vi "Obtain Hwnd and instantiate.vi"(0 "Py Doc in":refnum<class "Py Doc.lvclass">, 11 "error in (no error)":errorcluster) -> (4 "Document Out":refnum<class "Document.lvclass">, 6 "Document out":refnum<class "Document.lvclass">, 15 "error out":errorcluster)   [LabVIEW 2016, in "Py Doc.lvclass"]
uses:
  Py Doc.lvclass
  D:/Navin Workspace/MDI/source code/Document/Document base/Document.lvclass
  Document base/Document.lvclass
  Document base/Document.lvclass/Document.ctl
  Child Classes/Py Editor/Py Editor.lvclass
  Child Classes/Py Shell/Py Shell.lvclass
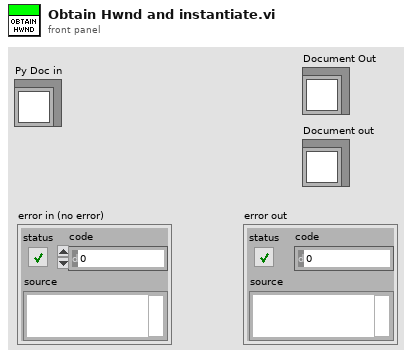
[diagram p1: front panel]
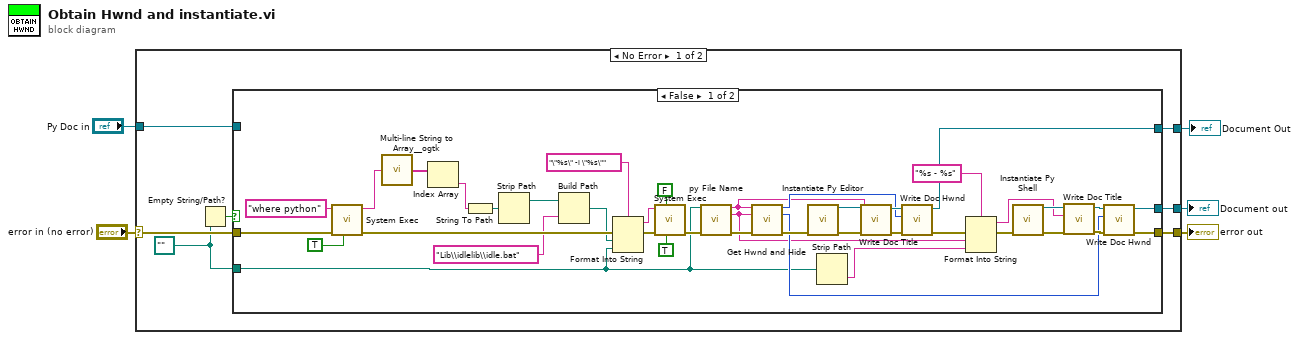
[diagram p0: block diagram]
diagram:
  n1 = case shown="No Error" "error in (no error)" {
    selector: "error in (no error)" -> [w11 w56]
    tunnel: "Py Doc in" -> [w10 w55]
    tunnel: [w12 w56] -> w4
    tunnel: [w8 w55] -> w2
    tunnel: [w7 w55] -> w1
    frame No Error {
      w6 = path "" ("Document Path")
      n2 = Empty String/Path?(string/path=w6) -> (empty?=w9:bool)
      n3 = case shown="False" w9 {
        tunnel: [w22 w54] -> w12
        tunnel: w11 -> [w35 w54]
        tunnel: w10 -> [_ w53]
        tunnel: w6 -> [w18 _]
        tunnel: [w20 w53] -> w8
        tunnel: [w19 w53] -> w7
        frame False {
          n4 = call <vilib>:"System Exec.vi"("run minimized? (F)"=TRUE, "error in (no error)"=w35, "command line"="where python") -> ("error out"=w52:errorcluster, "standard output"=w33:string)  [unwired: 5 in, 2 out]
          n5 = call <userlib>:"Multi-line String to Array__ogtk.vi"("string"=w33) -> ("lines"=w34:string[])
          n6 = Index Array(array=w34) -> (element=w32:string)  [unwired: 1 in]
          n7 = String To Path(string=w32) -> (path=w48:path)
          n8 = Strip Path(path=w48) -> (stripped path=w49:path)  [unwired: 1 out]
          n9 = Build Path(base path=w49, name or relative path="Lib\\idlelib\\idle.bat") -> (appended path=w51:path)
          n10 = Format Into String(format string="\"%s\" -i \"%s\"", error in=w52, w51, w18) -> (resulting string=w37:string, error out=w36:errorcluster)  [unwired: 1 in]
          n11 = call <vilib>:"System Exec.vi"("run minimized? (F)"=TRUE, "wait until completion? (T)"=FALSE, "error in (no error)"=w36, "command line"=w37) -> ("error out"=w42:errorcluster)  [unwired: 4 in, 3 out]
          n12 = call "py File Name.vi"("Path"=w18, "error in (no error)"=w42) -> ("Doc Name"=w43:string, "Shell Name"=w15:string, "error out"=w40:errorcluster)  [unwired: 11 in]
          n13 = call "Get Hwnd and Hide.vi"("Doc Name"=w43, "Shell Name"=w15, "error in (no error)"=w40) -> ("Child hwnd"=w44:u32, "Shell hwnd"=w21:u32, "error out"=w28:errorcluster)  [unwired: 10 in]
          n14 = call "Instantiate Py Editor.vi"("error in (no error)"=w28) -> ("Document.lvclass"=w26:refnum<class "Document.lvclass">, "error out"=w27:errorcluster)  [unwired: 13 in]
          n15 = Strip Path(path=w18) -> (name=w14:string)  [unwired: 1 out]
          n16 = call "Write Doc Title.vi"("error in (no error)"=w27, "Doc Name"=w43, "Document in"=w26) -> ("error out"=w46:errorcluster, "Document out"=w45:refnum<class "Document.lvclass">)  [unwired: 7 in]
          n17 = call "Write Doc Hwnd.vi"("error in (no error)"=w46, "Child Hwnd"=w44, "Document in"=w45) -> ("error out"=w23:errorcluster, "Document out"=w19:refnum<class "Document.lvclass">)  [unwired: 7 in]
          n18 = Format Into String(format string="%s - %s", error in=w23, w15, w14) -> (resulting string=w16:string, error out=w17:errorcluster)  [unwired: 1 in]
          n19 = call "Instantiate Py Shell.vi"("error in (no error)"=w17) -> ("Document.lvclass"=w29:refnum<class "Document.lvclass">, "error out"=w25:errorcluster)  [unwired: 13 in]
          n20 = call "Write Doc Title.vi"("error in (no error)"=w25, "Doc Name"=w16, "Document in"=w29) -> ("error out"=w24:errorcluster, "Document out"=w30:refnum<class "Document.lvclass">)  [unwired: 7 in]
          n21 = call "Write Doc Hwnd.vi"("error in (no error)"=w24, "Child Hwnd"=w21, "Document in"=w30) -> ("error out"=w22:errorcluster, "Document out"=w20:refnum<class "Document.lvclass">)  [unwired: 7 in]
        }
        frame True {
        }
      }
    }
    frame Error {
    }
  }
  "error out" <- w4
  "Document out" <- w2
  "Document Out" <- w1
